vi "get active handles.vi"(8 "error in (no error)":errorcluster, 10 "Return All?":bool, 11 "Camera in":refnum<class "Camera.lvclass">) -> (0 "error out":errorcluster, 1 "Active Cameras":T1[](array[typedef]), 2 "Handles":variant[](array[variant]), 3 "Camera out":refnum<class "Camera.lvclass">, 5 "Camera Names":string[](array[string]))   [LabVIEW 2022 SP3, in "Camera.lvlib" / "Camera.lvclass"]
uses:
  Camera.lvclass
  Resources/Type Defs/Physical Camera Assignment.ctl
  Camera.lvclass/Camera.ctl
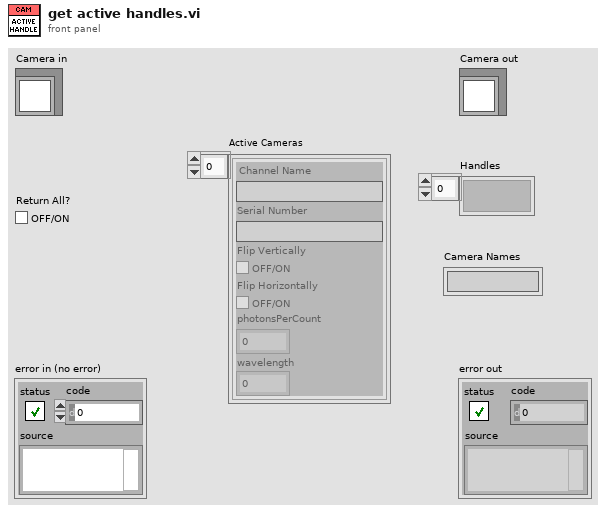
[diagram p1: front panel]
types:
  T1 = typedef "Physical Camera Assignment.ctl" = cluster{"Channel Name":string, "Serial Number":string, "Flip Vertically":bool, "Flip Horizontally":bool, "photonsPerCount":dbl, "wavelength":i16}
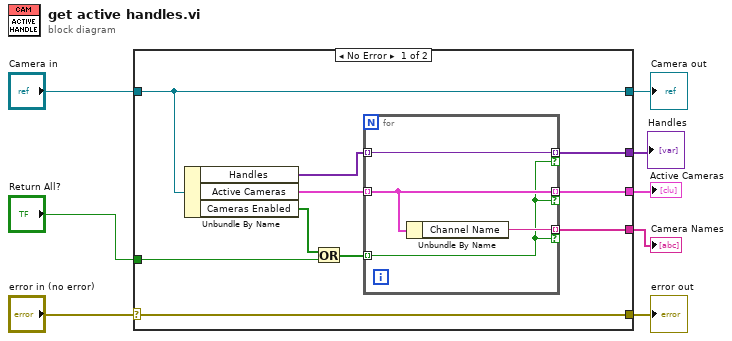
[diagram p0: block diagram]
diagram:
  n1 = case shown="No Error" "error in (no error)" {
    selector: "error in (no error)" -> [w18 w24]
    tunnel: [w18 w24] -> w7
    tunnel: [w12 w23] -> w5
    tunnel: "Camera in" -> [w12 w23]
    tunnel: [w15 _] -> w4
    tunnel: [w14 _] -> w3
    tunnel: [w13 _] -> w2
    tunnel: "Return All?" -> [w9 _]
    frame No Error {
      n2 = Unbundle By Name(w12) -> ("Handles"=w17:variant[], "Active Cameras"=w16:T1[], "Cameras Enabled"=w10:bool[])
      n3 = Or(x=w10, y=w9) -> (x .or. y?=w11:bool[])
      n4 = for {
        tunnel: w17 -> [w22] mode=indexing
        tunnel: w16 -> [w21] mode=indexing
        tunnel: w11 -> [w19] mode=indexing
        tunnel: [w21] -> w14 mode=indexing if=w19
        tunnel: [w22] -> w15 mode=indexing if=w19
        tunnel: [w20] -> w13 mode=indexing if=w19
        n5 = Unbundle By Name(w21) -> ("Channel Name"=w20:string)
      }
    }
    frame Error {
    }
  }
  "error out" <- w7
  "Camera out" <- w5
  "Active Cameras" <- w3
  "Camera Names" <- w2
  "Handles" <- w4
